vi "Online_TRAC_Calculate.vi"(8 "error in (no error)":errorcluster, 11 "Online_TRAC in":refnum<class "Online_TRAC.lvclass">) -> (0 "error out":errorcluster, 3 "Online_TRAC out":refnum<class "Online_TRAC.lvclass">)   [LabVIEW 2021, in "Online_TRAC.lvclass"]
uses:
  Online_TRAC.lvclass
  Online_TRAC.lvclass/Online_TRAC.ctl
  Read Square Cross Sum.vi
  Read Square Esitmated Sum.vi
  Read Square True Sum.vi
  Write TRAC.vi
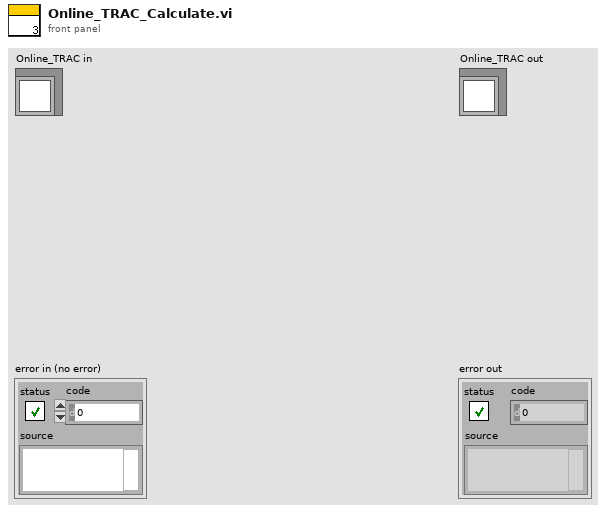
[diagram p1: front panel]
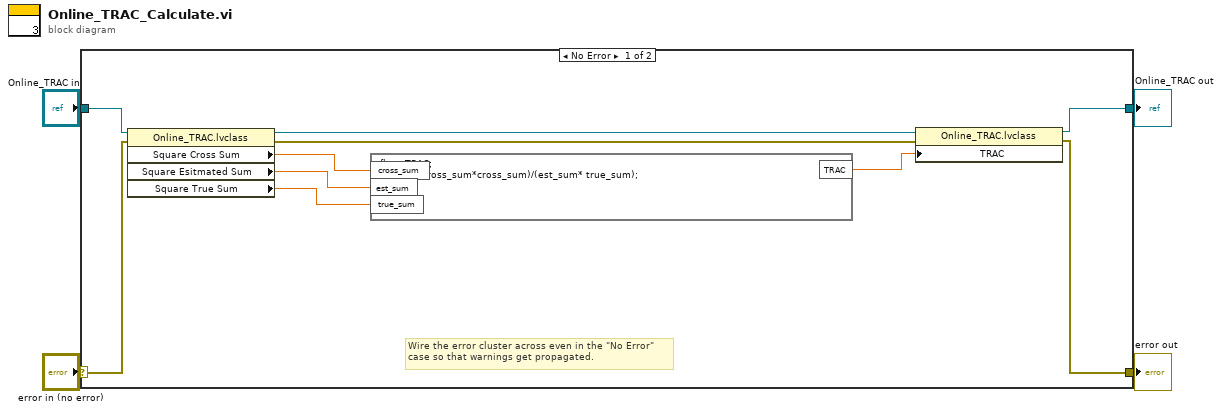
[diagram p0: block diagram]
diagram:
  n1 = case shown="No Error" "error in (no error)" {
    selector: "error in (no error)" -> [w6 w16]
    tunnel: [w5 w16] -> w3
    tunnel: [w8 w15] -> w2
    tunnel: "Online_TRAC in" -> [w7 w15]
    frame No Error {
      # "Wire the error cluster across even in the \"No Error\"\ncase so that warnings get propagated."
      n2 = property class="Online_TRAC.lvclass"(reference=w7, error in=w6) -> (reference out=w10:refnum<class "Online_TRAC.lvclass">, error out=w9:errorcluster, "Square Cross Sum"=w14:dbl, "Square Esitmated Sum"=w13:dbl, "Square True Sum"=w12:dbl)
      n3 = formula code="float TRAC;\nTRAC = (cross_sum*cross_sum)/(est_sum* true_sum);"("cross_sum"=w14, "est_sum"=w13, "true_sum"=w12) -> ("TRAC"=w11:dbl)
      n4 = property class="Online_TRAC.lvclass"(reference=w10, error in=w9, "TRAC"=w11) -> (reference out=w8:refnum<class "Online_TRAC.lvclass">, error out=w5:errorcluster)
    }
    frame Error {
    }
  }
  "error out" <- w3
  "Online_TRAC out" <- w2
